vi "Motor tester.vi"() -> ()   [LabVIEW 2017]
uses:
  <vilib>/addons/eal4LabVIEW/ApiLib/Connection control/ealApiConnect_string.vi
  <vilib>/addons/eal4LabVIEW/ApiLib/Connection control/ealApiInitialise_int.vi
  <vilib>/addons/eal4LabVIEW/eal4LabVIEW.lvlib
panel:
  out "diagnosis text 2":string
  out "diagnosis text 3":string
  out "diagnosis text":string
  out "error out":errorcluster
  out "name":string
  in  "ip address":string
  in  "parameters set":T1
  out "getActualPosition":dbl
  in  "stop":bool
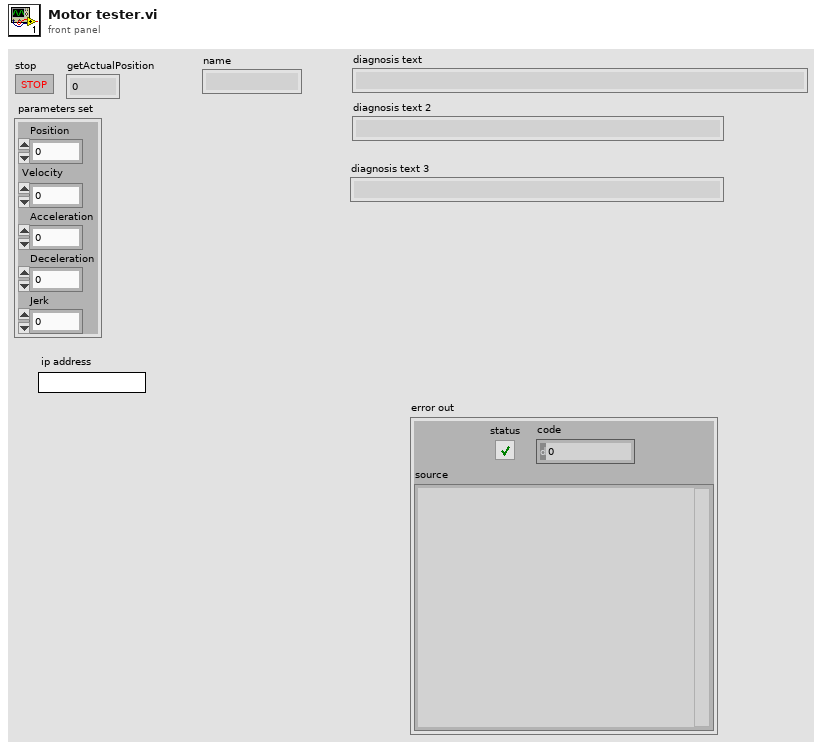
[diagram p1: front panel]
types:
  T1 = cluster{"Position":dbl, "Velocity":dbl, "Acceleration":dbl, "Deceleration":dbl, "Jerk":dbl}
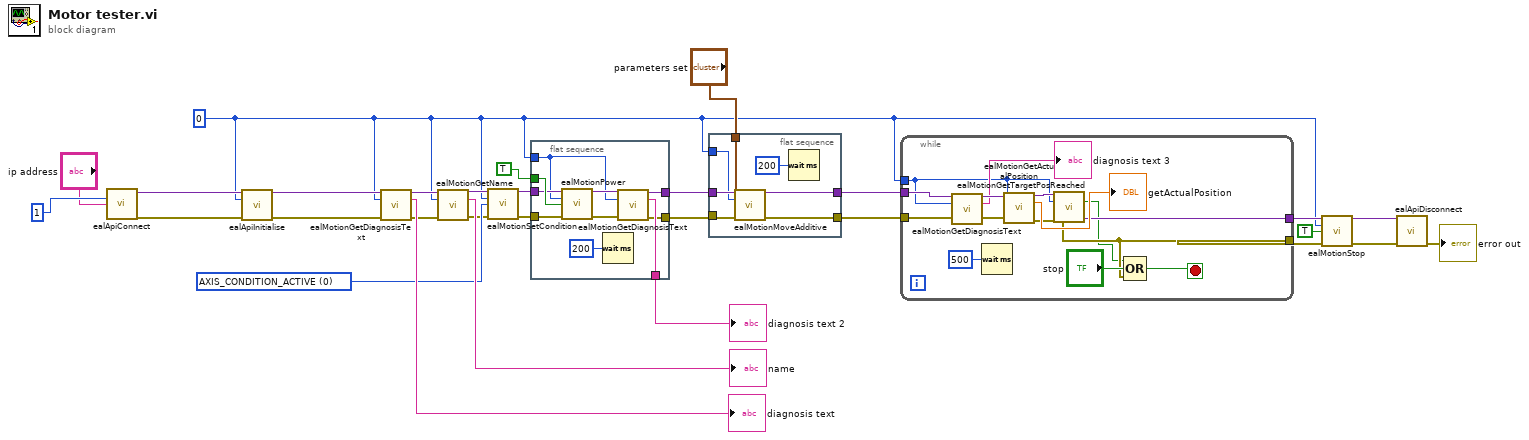
[diagram p0: block diagram]
diagram:
  w13 = 0 items=["AXIS_CONDITION_ACTIVE"=0, "AXIS_CONDITION_PARKING"=1, "AXIS_CONDITION_DEACTIVATED"=2, "AXIS_CONDITION_ACTIVE_DECOUPLED"=4, "AXIS_CONDITION_PARKING_DECOUPLED"=5, "AXIS_CONDITION_DEACTIVATED_DECOUPLED"=6, "AXIS_CONDITION_ACTIVE_PARAMETERIZATION"=8, "AXIS_CONDITION_PARKING_PARAMETERIZATION"=9, "AXIS_CONDITION_DEACTIVATED_PARAMETERIZATION"=10, "AXIS_CONDITION_ACTIVE_DECOUPLED_PARAMETERIZATION"=12, "AXIS_CONDITION_PARKING_DECOUPLED_PARAMETERIZATION"=13, "AXIS_CONDITION_DEACTIVATED_DECOUPLED_PARAMETERIZATION"=14] ("condition")
  w1 = 0 ("slave index")
  n1 = call-poly <vilib>:"ealApiConnect.vi"("maximum no of axes"=1, "ip address"="ip address") -> ("connection out"=w21:variant, "error out"=w2:errorcluster)  [unwired: 12 in]
  n2 = call-poly <vilib>:"ealApiInitialise.vi"("connection in"=w21, "slave index"=w1, "error in (no error)"=w2) -> ("connection out"=w7:variant, "error out"=w6:errorcluster)  [unwired: 11 in]
  n3 = call <vilib>:"ealMotionGetDiagnosisText.vi"("connection in"=w7, "slave index"=w1, "error in (no error)"=w6) -> ("connection out"=w19:variant, "diagnosis text"=→"diagnosis text":string, "error out"=w5:errorcluster)  [unwired: 10 in]
  n4 = call <vilib>:"ealMotionGetName.vi"("connection in"=w19, "slave index"=w1, "error in (no error)"=w5) -> ("connection out"=w20:variant, "name"=→"name":string, "error out"=w3:errorcluster)  [unwired: 10 in]
  n5 = call <vilib>:"ealMotionSetCondition.vi"("connection in"=w20, "slave index"=w1, "condition"=w13, "error in (no error)"=w3) -> ("connection out"=w14:variant, "error out"=w4:errorcluster)  [unwired: 10 in]
  n6 = flat-sequence {
    tunnel: TRUE ("value") -> [w39]
    tunnel: w14 -> [w38]
    tunnel: w4 -> [w37]
    tunnel: [w35] -> w17
    tunnel: [w34] -> w16
    tunnel: w1 -> [w33]
    tunnel: [w31] -> w15
    frame #0 {
      n7 = call <vilib>:"ealMotionPower.vi"("connection in"=w38, "slave index"=w33, "value"=w39, "error in (no error)"=w37) -> ("connection out"=w36:variant, "error out"=w32:errorcluster)  [unwired: 10 in]
      n8 = Wait (ms)(milliseconds to wait=u32 200) -> ()  [unwired: 1 out]
      n9 = call <vilib>:"ealMotionGetDiagnosisText.vi"("connection in"=w36, "slave index"=w33, "error in (no error)"=w32) -> ("connection out"=w35:variant, "diagnosis text"=w34:string, "error out"=w31:errorcluster)  [unwired: 10 in]
    }
  }
  n10 = flat-sequence {
    tunnel: [w46] -> w27
    tunnel: [w45] -> w26
    tunnel: "parameters set" -> [w44]
    tunnel: w17 -> [w43]
    tunnel: w1 -> [w42]
    tunnel: w15 -> [w41]
    frame #0 {
      n11 = call <vilib>:"ealMotionMoveAdditive.vi"("connection in"=w43, "slave index"=w42, "parameters set"=w44, "error in (no error)"=w41) -> ("connection out"=w46:variant, "error out"=w45:errorcluster)  [unwired: 10 in]
      n12 = Wait (ms)(milliseconds to wait=u32 200) -> ()  [unwired: 1 out]
    }
  }
  n13 = while {
    tunnel: w27 -> [w57]
    tunnel: w1 -> [w48]
    tunnel: w26 -> [w56]
    tunnel: [w51] -> w22
    tunnel: [w49] -> w9
    stop <- w52 stop-if-true
    n14 = call <vilib>:"ealMotionGetDiagnosisText.vi"("connection in"=w57, "slave index"=w48) -> ("connection out"=w54:variant, "diagnosis text"=→"diagnosis text 3":string)  [unwired: 11 in, 1 out]
    n15 = Wait (ms)(milliseconds to wait=u32 500) -> ()  [unwired: 1 out]
    n16 = call <vilib>:"ealMotionGetActualPosition.vi"("connection in"=w54, "slave index"=w48, "error in (no error)"=w56) -> ("connection out"=w50:variant, "getActualPosition"=→"getActualPosition":dbl, "error out"=w51:errorcluster)  [unwired: 10 in]
    n17 = call <vilib>:"ealMotionGetTargetPosReached.vi"("connection in"=w50, "slave index"=w48) -> ("connection out"=w49:variant, "target position reached"=w47:bool)  [unwired: 11 in, 1 out]
    n18 = Compound Arithmetic op=OR(w47, "stop", w51) -> (w52:bool)
  }
  n19 = call <vilib>:"ealMotionStop.vi"("connection in"=w9, "slave index"=w1, "stop"=TRUE, "error in (no error)"=w22) -> ("connection out"=w10:variant, "error out"=w12:errorcluster)  [unwired: 10 in]
  n20 = call <vilib>:"ealApiDisconnect.vi"("connection in"=w10, "error in (no error)"=w12) -> ("error out"=→"error out":errorcluster)  [unwired: 13 in]
  "diagnosis text 2" <- w16
